vi "Make DLL Param(Read Profile Req).vi"(1 "Read Profile Req":T3 {"Profile Pos" items=["CURRENT", "OLDEST", "SPECIFY"]}) -> (0 "DLL Read Profile Req":T2 {"Profile Pos" items=["CURRENT", "OLDEST", "SPECIFY"]})   [LabVIEW 2015, in "KEYENCE LJ-X8000A.lvlib"]
uses:
  KEYENCE LJ-X8000A.lvlib
  Public/Clusters/Read Profile Req.ctl
  Public/Constants/Profile Pos.ctl
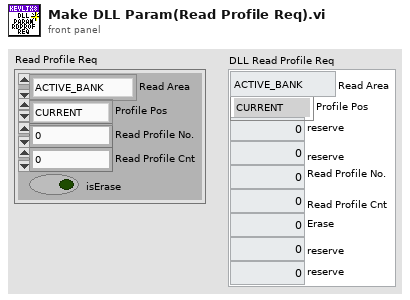
[diagram p1: front panel]
types:
  T1 = typedef "KEYENCE LJ-X8000A.lvlib/Profile Pos.ctl" = u8
  T2 = cluster{"Read Area":enum8{"ACTIVE_BANK", "INACTIVE_BANK"}, "Profile Pos":T1, "reserve":u8, "reserve":u8, "Read Profile No.":u32, "Read Profile Cnt":u8, "Erase":u8, "reserve":u8, "reserve":u8}
  T3 = typedef "KEYENCE LJ-X8000A.lvlib/Read Profile Req.ctl" = cluster{"Read Area":enum8{"ACTIVE_BANK", "INACTIVE_BANK"}, "Profile Pos":T1, "Read Profile No.":u32, "Read Profile Cnt":u8, "isErase":bool}
  T4 = cluster{"Read Area":enum8{"ACTIVE_BANK", "INACTIVE_BANK"}, "Profile Pos":T1, "reserve":u8, "reserve":u8, "Read Profile No.":u32, "Read Profile Cnt":u8, u8, "reserve":u8, "reserve":u8}
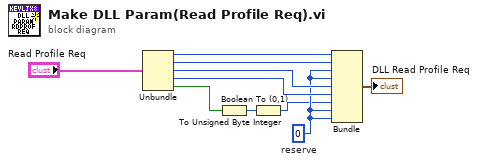
[diagram p0: block diagram]
diagram:
  w5 = u8 0  # reserve
  n1 = Unbundle("Read Profile Req") -> ("Read Area"=w2:enum8{"ACTIVE_BANK", "INACTIVE_BANK"}, "Profile Pos"=w9:T1, "Read Profile No."=w8:u32, "Read Profile Cnt"=w7:u8, "isErase"=w6:bool)
  n2 = Boolean To (0,1)(Boolean=w6) -> (0, 1=w4:i16)
  n3 = To Unsigned Byte Integer(number=w4) -> (unsigned 8bit integer=w3:u8)
  n4 = Bundle("Read Area"=w2, "Profile Pos"=w9, "reserve"=w5, "reserve"=w5, "Read Profile No."=w8, "Read Profile Cnt"=w7, w3, "reserve"=w5, "reserve"=w5) -> (→"DLL Read Profile Req":T4)  [unwired: 1 in]
